vi "Get_DT_Board_Info.vi"() -> (1 "DT Cluster Array":T1[](array[typedef]))   [LabVIEW 2013]
uses:
  Controls/DT_Cluster.ctl
  Controls/DT_Mode.ctl
  Globals/Meas_global.vi
  <userlib>/LV-Link3/PolySubVIs/DtCreateDinChan.vi
  <userlib>/LV-Link3/PolySubVIs/DtOLReadSingle.vi
panel:
  out "Array 6":i32[](array[numeric])
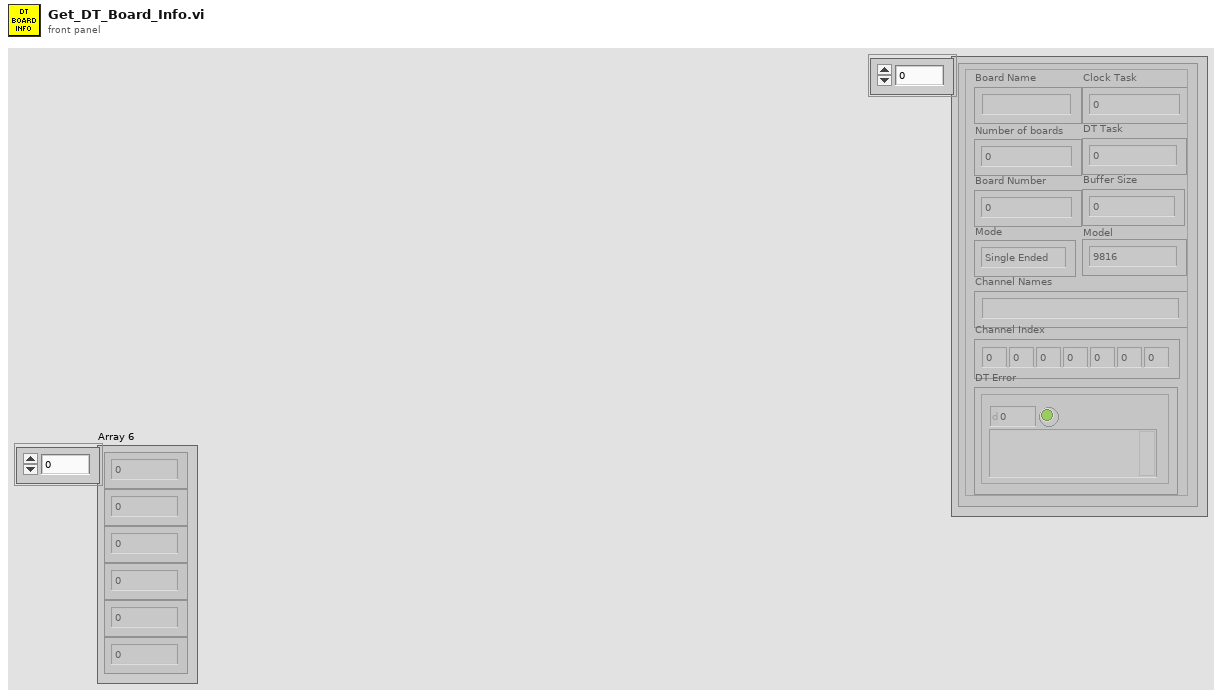
[diagram p1: front panel]
types:
  T1 = typedef "DT_Cluster.ctl" = cluster{"Board Name":string, "Number of boards":u32, "Board Number":u32, "Channel Names":string, "Channel Index":i32[], "DT Task":i32, "DT Error":errorcluster, "Mode":T2, "Buffer Size":u32, "Clock Task":i32, "Model":enum16{"9816", "9836", "9853"}}
  T2 = typedef "DT_Mode.ctl" = enum16{"Single Ended", "Differential"}
  T3 = typedef "Ch_and_Spans.ctl" = cluster{"high limit (10V)":sgl, "low limit (-10V)":sgl, "Ch No":i16, "Var name":string, "Use Latest Calib":bool}
  T4 = cluster{"Board Number":u32, "Data Translation Board Cluster":T1}
  T5 = cluster{"Board Number":u32, "Data Translation Board Cluster":T1}[]
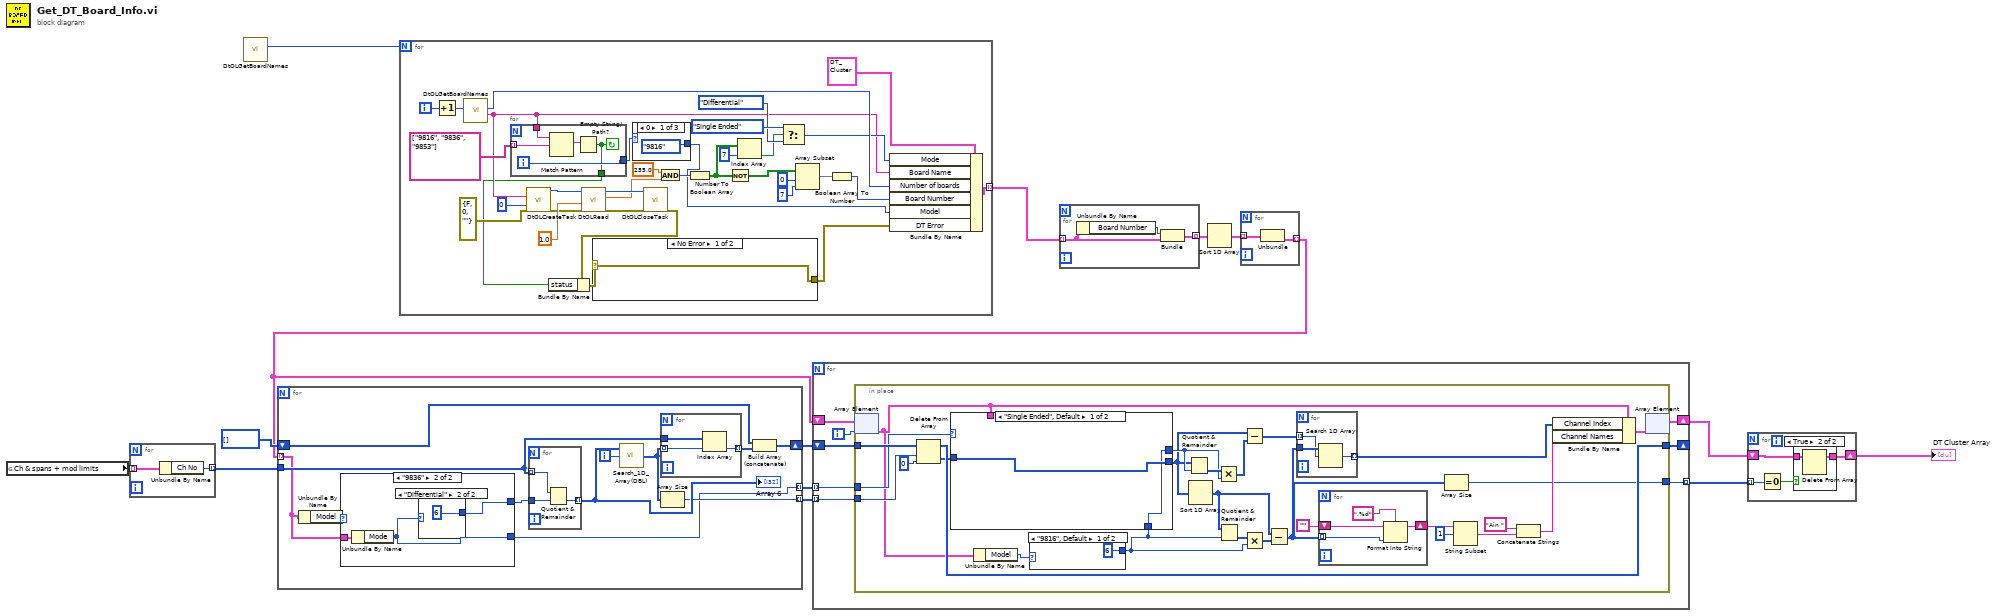
[diagram p0: block diagram]
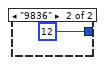
[diagram p3: hidden frame]
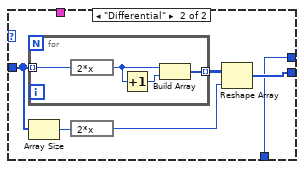
[diagram p4: hidden frame]
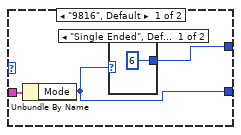
[diagram p5: hidden frame]
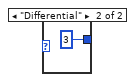
[diagram p6: hidden frame]
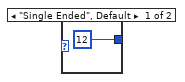
[diagram p7: hidden frame]
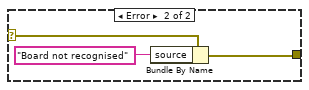
[diagram p8: hidden frame]
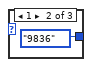
[diagram p9: hidden frame]
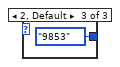
[diagram p10: hidden frame]
diagram:
  n1 = global read "Meas_global.vi" "Ch & spans + mod limits"() -> (w7:T3[])
  n2 = for {
    tunnel: w7 -> [w16] mode=indexing
    tunnel: [w15] -> w6 mode=indexing
    n3 = Unbundle By Name(w16) -> ("Ch No"=w15:i16)
  }
  n4 = call <userlib>:"DtOLGetBoardNames.vi"() -> ("Number of boards"=w14:u32)  [unwired: 9 in, 2 out]
  n5 = for {
    N: w14 -> [_]
    tunnel: [w36] -> w13 mode=indexing
    i -> [w50]
    n6 = Increment(x=w50) -> (x+1=w49:i32)
    n7 = call <userlib>:"DtOLGetBoardNames.vi"("Select Board"=w49) -> ("Board Name"=w23:string, "Number of boards"=w39:u32)  [unwired: 8 in, 1 out]
    n8 = for {
      tunnel: string[] ["9816", "9836", "9853"] -> [w62] mode=indexing
      tunnel: w23 -> [w61]
      tunnel: [w59] -> w22
      tunnel: [w58] -> w19
      i -> [w59]
      stop <- w58 continue-if-true
      n9 = Match Pattern(string=w61, regular expression=w62) -> (match substring=w60:string)  [unwired: 1 in, 3 out]
      n10 = Empty String/Path?(string/path=w60) -> (empty?=w58:bool)
    }
    n11 = call-poly <userlib>:"DtOLCreateTask.vi"("Board Name"=w23, "Port Number"=u32 0, "error in (no error)"=errorcluster {"status"=FALSE, "code"=0, "source"=""} ("Error Out")) -> ("Task out"=w47:i32, "error out"=w44:errorcluster)  [unwired: 11 in]
    n12 = call-poly <userlib>:"DtOLRead.vi"("error in (no error)"=w44, "Timeout"=1.0 ("Samples Per Channel"), "Task in"=w47) -> ("error out"=w43:errorcluster, "Data Out"=w28:dbl, "Task out"=w42:i32)  [unwired: 6 in]
    n13 = case shown="0" w22 {
      tunnel: [enum16{"9816", "9836", "9853"}."9816" ("Model") enum16{"9816", "9836", "9853"}."9836" ("Model") enum16{"9816", "9836", "9853"}."9853" ("Model")] -> w21
      frame 0 {
      }
      frame 1 {
      }
      frame 2, Default {
      }
    }
    n14 = call <userlib>:"DtOLCloseTask.vi"("Error in"=w43, "Task in"=w42) -> ("Error Out"=w18:errorcluster)  [unwired: 9 in]
    n15 = Bundle By Name(cluster=w18, "status"=w19) -> (w20:errorcluster)
    n16 = case shown="No Error" w20 {
      selector: w20 -> [w51 w54]
      tunnel: [w51 w52] -> w17
      frame No Error {
      }
      frame Error {
        n17 = Bundle By Name(cluster=w54, "source"="Board not recognised") -> (w52:errorcluster)
      }
    }
    n18 = And(x=255.0, y=w28) -> (x .and. y?=w45:i32)
    n19 = Number To Boolean Array(number=w45) -> (Boolean array=w35:bool[])
    n20 = Not(x=w35) -> (.not. x?=w32:bool[])
    n21 = Index Array(array=w35, index=7) -> (element=w33:bool)
    n22 = Select(t=DT_Mode."Single Ended" ("Mode"), s=w33, f=DT_Mode."Differential") -> (s? t:f=w29:T2)
    n23 = Array Subset(array=w32, index=0, length=7) -> (w27:bool[])
    n24 = Boolean Array To Number(Boolean array=w27) -> (number=w25:u32)
    n25 = Bundle By Name(cluster=T1 {"Board Name"="", "Number of boards"=0, "Board Number"=0, "Channel Names"="", "Channel Index"=[], "DT Task"=0, "DT Error"={"status"=FALSE, "code"=0, "source"=""}, "Mode"=enum."Single Ended", "Buffer Size"=0, "Clock Task"=0, "Model"=enum."9816"} ("Data Translation Board Cluster"), "Mode"=w29, "Board Name"=w23, "Number of boards"=w39, "Board Number"=w25, "Model"=w21, "DT Error"=w17) -> (w36:T1)
  }
  n26 = for {
    tunnel: w13 -> [w65] mode=indexing
    tunnel: [w63] -> w12 mode=indexing
    n27 = Unbundle By Name(w65) -> ("Board Number"=w64:u32)
    n28 = Bundle("Board Number"=w64, "Data Translation Board Cluster"=w65) -> (w63:T4)  [unwired: 1 in]
  }
  n29 = Sort 1D Array(array=w12) -> (sorted array=w11:T5)
  n30 = for {
    tunnel: w11 -> [w67] mode=indexing
    tunnel: [w66] -> w4 mode=indexing
    n31 = Unbundle(w67) -> ("Data Translation Board Cluster"=w66:T1)  [unwired: 1 out]
  }
  n32 = for {
    tunnel: w6 -> [w72]
    tunnel: [w76] -> w10 mode=indexing
    shift-right: [w74] -> w8
    shift-left: i32[] [] -> [w73]
    tunnel: w4 -> [w69] mode=indexing
    tunnel: [w70] -> w5 mode=indexing
    i -> [w79]
    n33 = Unbundle By Name(w69) -> ("Model"=w68:enum16{"9816", "9836", "9853"})
    n34 = case shown="\"9836\"" w68 {
      tunnel: [w82 w87] -> w71
      tunnel: w69 -> [w81 w86]
      tunnel: [w80 w85] -> w70
      frame "9816", Default {
        n35 = Unbundle By Name(w81) -> ("Mode"=w80:T2)
        n36 = case shown="\"Single Ended\", Default" w80 {
          tunnel: [6 ("y") 3 ("y")] -> w82
          frame "Single Ended", Default {
          }
          frame "Differential" {
          }
        }
      }
      frame "9836" {
        n37 = Unbundle By Name(w86) -> ("Mode"=w85:T2)
        n38 = case shown="\"Differential\"" w85 {
          tunnel: [12 ("y") 6 ("y")] -> w87
          frame "Single Ended", Default {
          }
          frame "Differential" {
          }
        }
      }
    }
    n39 = for {
      tunnel: w72 -> [w94] mode=indexing
      tunnel: [w95] -> w78 mode=indexing
      tunnel: w71 -> [w93]
      n40 = Quotient & Remainder(x=w94, y=w93) -> (floor(x/y)=w95:i32)  [unwired: 1 out]
    }
    "Array 6" <- w78
    n41 = call "Search_1D_Array(DBL).vi"("Array"=w78, "Element Data"=w79) -> ("Indicies of Elements"=w77:i32[])  [unwired: 6 in, 1 out]
    n42 = for {
      tunnel: w77 -> [w91] mode=indexing
      tunnel: w72 -> [w92]
      tunnel: [w90] -> w75 mode=indexing
      n43 = Index Array(array=w92, index=w91) -> (element=w90:i16)
    }
    n44 = Array Size(array=w77) -> (size(s)=w76:i32)
    n45 = Build Array (concatenate)(w73, w75) -> (w74:i32[])
  }
  n46 = for {
    tunnel: w10 -> [w102] mode=indexing
    shift-right: [w101] -> _
    shift-left: w8 -> [w103]
    shift-right: [w98] -> w2
    shift-left: w4 -> [w99]
    tunnel: w5 -> [w100] mode=indexing
    tunnel: [w96] -> w3 mode=indexing
    i -> [w97]
    n47 = in-place {
      in-place-border: w103 -> [w130]
      in-place-border: w102 -> [w129]
      in-place-border: [w123] -> w101
      in-place-border: w100 -> [w112]
      in-place-border: [w107] -> w96
      n48 = in-place-array #1(w99, w97) -> (w105:T1)
      n49 = Delete From Array(array=w130, length=w129, index=0) -> (deleted portion=w121:i32[], array with subset deleted=w123:i32[])
      n50 = Unbundle By Name(w105) -> ("Model"=w106:enum16{"9816", "9836", "9853"})
      n51 = case shown="\"9816\", Default" w106 {
        tunnel: [6 ("offset (0)") 12 ("offset (0)")] -> w104
        frame "9816", Default {
        }
        frame "9836" {
        }
      }
      n52 = case shown="\"Single Ended\", Default" w112 {
        tunnel: w121 -> [w134 w137]
        tunnel: [w133 w135] -> w115
        tunnel: [w134 w136] -> w113
        tunnel: w105 -> [_ _]
        tunnel: w104 -> [w133 w135]
        frame "Single Ended", Default {
        }
        frame "Differential" {
          n53 = for {
            tunnel: [w143] -> w139 mode=indexing
            tunnel: w137 -> [w141] mode=indexing
            n54 = expression code="2*x"(w141) -> (w142:i32)
            n55 = Increment(x=w142) -> (x+1=w144:i32)
            n56 = Build Array(w142, w144) -> (w143:i32[])
          }
          n57 = Array Size(array=w137) -> (size(s)=w140:i32)
          n58 = expression code="2*x"(w140) -> (w138:i32)
          n59 = Reshape Array(w139, w138) -> (w136:i32[])
        }
      }
      n60 = Quotient & Remainder(x=w113, y=w115) -> (floor(x/y)=w117:i32[])  [unwired: 1 out]
      n61 = Sort 1D Array(array=w113) -> (sorted array=w118:i32[])
      n62 = Multiply(x=w117, y=w115) -> (x*y=w116:i32[])
      n63 = Quotient & Remainder(x=w118, y=w104) -> (floor(x/y)=w119:i32[])  [unwired: 1 out]
      n64 = Subtract(x=w113, y=w116) -> (x-y=w114:i32[])
      n65 = Multiply(x=w119, y=w104) -> (x*y=w120:i32[])
      n66 = Subtract(x=w118, y=w120) -> (x-y=w108:i32[])
      n67 = for {
        tunnel: w108 -> [w151]
        tunnel: w114 -> [w150] mode=indexing
        tunnel: [w149] -> w110 mode=indexing
        n68 = Search 1D Array(1D array=w151, element=w150) -> (index of element=w149:i32)  [unwired: 1 in]
      }
      n69 = for {
        shift-right: [w146] -> w128
        shift-left: "" -> [w147]
        tunnel: w108 -> [w145] mode=indexing
        n70 = Format Into String(format string=",%d", initial string=w147, w145) -> (resulting string=w146:string)  [unwired: 1 in, 1 out]
      }
      n71 = Array Size(array=w108) -> (size(s)=w107:i32)
      n72 = String Subset(string=w128, offset (0)=1) -> (substring=w125:string)  [unwired: 1 in]
      n73 = Concatenate Strings("Ain ", w125) -> (w109:string)
      n74 = Bundle By Name(cluster=w105, "Channel Index"=w110, "Channel Names"=w109) -> (w111:T1)
      n75 = in-place-array #1(w111) -> (w98:T1[])  [unwired: 1 out]
    }
  }
  n76 = for {
    tunnel: w3 -> [w155] mode=indexing
    shift-right: [w152] -> w1
    shift-left: w2 -> [w154]
    n77 = Equal To 0?(x=w155) -> (x = 0?=w153:bool)
    n78 = case shown="True" w153 {
      tunnel: w154 -> [w156 w158]
      tunnel: [w156 w157] -> w152
      frame False {
      }
      frame True {
        n79 = Delete From Array(array=w158) -> (array with subset deleted=w157:T1[])  [unwired: 2 in, 1 out]
      }
    }
  }
  "DT Cluster Array" <- w1
